vi "Recursive file list.vi"(8 "error in (no error)":errorcluster, 10 "Path":string, 11 "WebDAV in":refnum<class "WebDAV.lvclass">) -> (0 "error out":errorcluster, 1 "Files":string[](array[string]), 2 "Directories":string[](array[string]), 3 "WebDAV out":refnum<class "WebDAV.lvclass">)   [LabVIEW 2015, in "RT Management.lvlib" / "WebDAV.lvclass"]
uses:
  WebDAV.lvclass
  WebDAV.lvclass/WebDAV.ctl
  Get Session.vi
  <vilib>/Utility/error.llb/Trim Whitespace.vi
  File Transfer Behavior/File Transfer Behavior.lvclass
  <vilib>/WebDAVClient/NI_WebDAV.lvlib
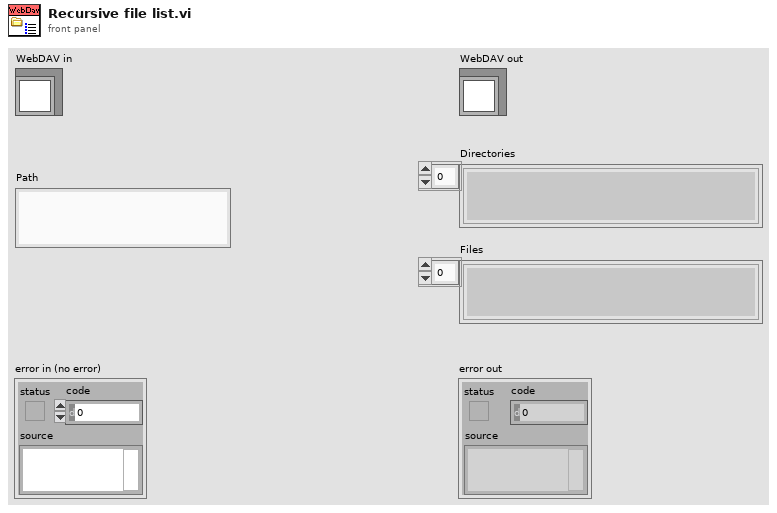
[diagram p1: front panel]
types:
  T1 = typedef "NI_WebDAV.lvlib/SessionHandle.ctl" = refnum<k1>
  T2 = typedef "NI_WebDAV.lvlib/FileInfo.ctl" = cluster{"type":string, "size":u64, "last modification":timestamp, "display name":string, "uri":string}
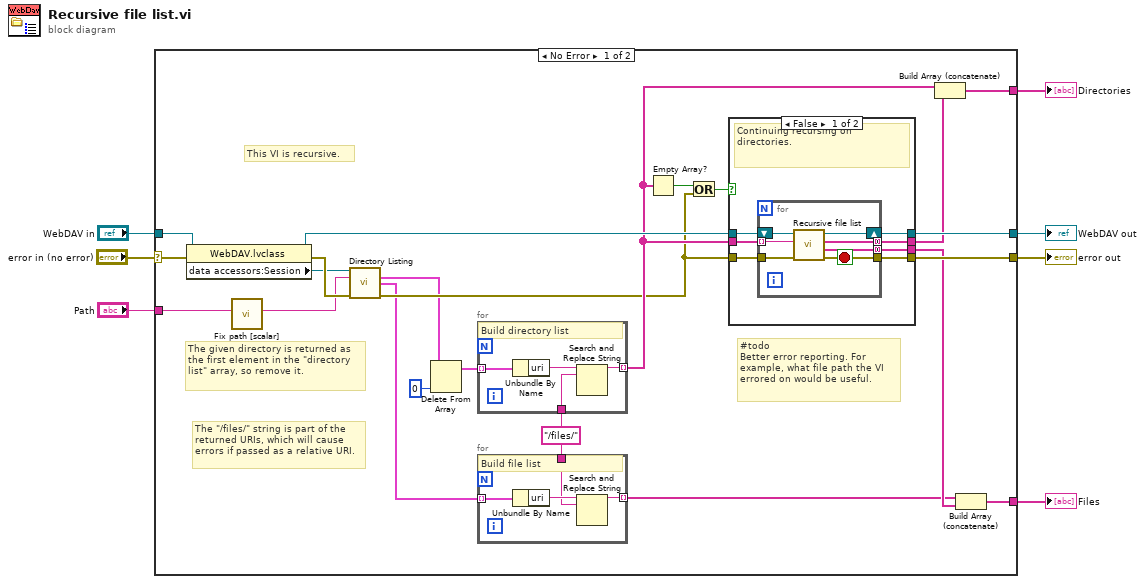
[diagram p0: block diagram]
diagram:
  n1 = case shown="No Error" "error in (no error)" {
    selector: "error in (no error)" -> [w22 w56]
    tunnel: [w30 w56] -> w6
    tunnel: [w27 w55] -> w5
    tunnel: "WebDAV in" -> [w29 w55]
    tunnel: "Path" -> [w9 _]
    tunnel: [w25 _] -> w2
    tunnel: [w23 _] -> w3
    frame No Error {
      w16 = "/files/" ("search string")
      # "#todo\nBetter error reporting. For example, what file path the VI errored on would be useful."
      # "This VI is recursive."
      # "The \"/files/\" string is part of the returned URIs, which will cause errors if passed as a relative URI."
      # "The given directory is returned as the first element in the \"directory list\" array, so remove it."
      n2 = property class="WebDAV.lvclass"(reference=w29, error in=w22) -> (reference out=w28:refnum<class "WebDAV.lvclass">, error out=w21:errorcluster, "data accessors:Session"=w20:T1)
      n3 = call "Fix path [scalar].vi"("Path in"=w9) -> ("Path out"=w8:string)  [unwired: 8 in, 2 out]
      n4 = call <vilib>:"Directory Listing.vi"("session handle"=w20, "relative uri"=w8, "error in (no error)"=w21) -> ("directory list"=w10:T2[], "file list"=w11:T2[], "error out"=w14:errorcluster)  [unwired: 9 in, 1 out]
      n5 = Delete From Array(array=w10, index=0) -> (array with subset deleted=w17:T2[])  [unwired: 1 in, 1 out]
      n6 = for {
        tunnel: w17 -> [w38] mode=indexing
        tunnel: [w36] -> w19 mode=indexing
        tunnel: w16 -> [w35]
        # "Build directory list"
        n7 = Unbundle By Name(w38) -> ("uri"=w37:string)
        n8 = Search and Replace String(input string=w37, search string=w35) -> (result string=w36:string)  [unwired: 6 in, 3 out]
      }
      n9 = for {
        tunnel: w11 -> [w34] mode=indexing
        tunnel: [w32] -> w15 mode=indexing
        tunnel: w16 -> [w31]
        # "Build file list"
        n10 = Unbundle By Name(w34) -> ("uri"=w33:string)
        n11 = Search and Replace String(input string=w33, search string=w31) -> (result string=w32:string)  [unwired: 6 in, 3 out]
      }
      n12 = Empty Array?(array=w19) -> (empty?=w13:bool)
      n13 = Or(x=w13, y=w14) -> (x .or. y?=w12:bool)
      n14 = case shown="False" w12 {
        tunnel: [w39 w53] -> w30
        tunnel: w14 -> [w45 w53]
        tunnel: w28 -> [w44 w54]
        tunnel: [w43 w54] -> w27
        tunnel: [w42 _] -> w26
        tunnel: [w41 _] -> w24
        tunnel: w19 -> [w40 _]
        frame False {
          # "Continuing recursing on directories."
          n15 = for {
            tunnel: [w49] -> w42 mode=concatenating
            tunnel: [w48] -> w41 mode=concatenating
            tunnel: w40 -> [w47] mode=indexing
            tunnel: w45 -> [w52]
            tunnel: [w46] -> w39
            shift-right: [w50] -> w43
            shift-left: w44 -> [w51]
            stop <- w46 stop-if-true
            n16 = call-dynamic "Recursive file list.vi"("error in (no error)"=w52, "Path"=w47, "WebDAV in"=w51) -> ("error out"=w46:errorcluster, "Files"=w49:string[], "Directories"=w48:string[], "WebDAV out"=w50:refnum<class "WebDAV.lvclass">)  [unwired: 5 in]
          }
        }
        frame True {
          # "Directory array is empty or an error occurred. Stop recursion."
        }
      }
      n17 = Build Array (concatenate)(w19, w24) -> (w23:string[])
      n18 = Build Array (concatenate)(w15, w26) -> (w25:string[])
    }
    frame Error {
    }
  }
  "error out" <- w6
  "WebDAV out" <- w5
  "Files" <- w2
  "Directories" <- w3
